vi "Digitizer Sample Rate.vi"(8 "error in (no error)":errorcluster, 9 "Sample Rate (100000)":u32=100000, 10 "Digitize Function (Voltage)":u16(ring) items=["Digitize Voltage", "Digitize Current"], 11 "VISA resource name":refnum<visa-resource-name>="USB0::0x05E6::0x2461::04090176::INSTR") -> (0 "error out":errorcluster, 3 "VISA resource name out":refnum<visa-resource-name>="USB0::0x05E6::0x2461::04090176::INSTR")   [LabVIEW 2015, in "Keithley 2450.lvlib"]
doc: "This command defines the precise acquisition rate at which the digitizing measurements are made.\n\n<B>The Digitizer Voltage and Digitizer Current functions are only compatible with the 2461.</B>"
uses:
  <instrlib>/Keithley 2450/Keithley 2450.lvlib
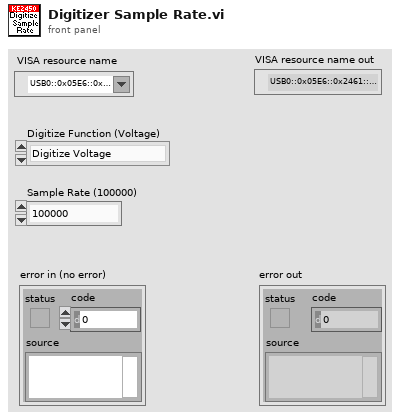
[diagram p1: front panel]
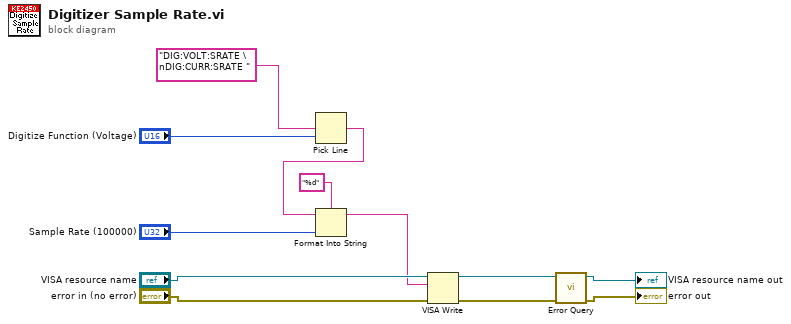
[diagram p0: block diagram]
diagram:
  n1 = Pick Line(multi-line string="DIG:VOLT:SRATE \nDIG:CURR:SRATE ", line index="Digitize Function (Voltage)") -> (output string=w2:string)  [unwired: 1 in]
  n2 = Format Into String(format string="%d", initial string=w2, "Sample Rate (100000)") -> (resulting string=w6:string)  [unwired: 1 in, 1 out]
  n3 = VISA Write(VISA resource name="VISA resource name", write buffer=w6, error in (no error)="error in (no error)") -> (VISA resource name out=w9:refnum<visa-resource-name>, error out=w8:errorcluster)  [unwired: 1 out]
  n4 = call <instrlib>:"Error Query.vi"("error in (no error)"=w8, "VISA resource name"=w9) -> ("error out"=→"error out":errorcluster, "VISA resource name out"=→"VISA resource name out":refnum<visa-resource-name>)  [unwired: 8 out]
